vi "Populate Ring.vi"(5 "Sort Alphabetically instead of by Hierarchy?(T)":bool=TRUE, 7 "Close Reference?(T)":bool=TRUE, 8 "error in (no error)":errorcluster, 10 "Hierarchy Filter(empty=all)":string, 11 "Ring in":refnum<vi>) -> (0 "error out":errorcluster, 1 "Success?":bool, 3 "Classes found":string[](array[string]))   [LabVIEW 2020, in "ClassLoader.lvlib"]
doc: "Populate a ring control with a the hierarchy loaded using the given Hierarchy Filter."
uses:
  ClassLoader.lvlib
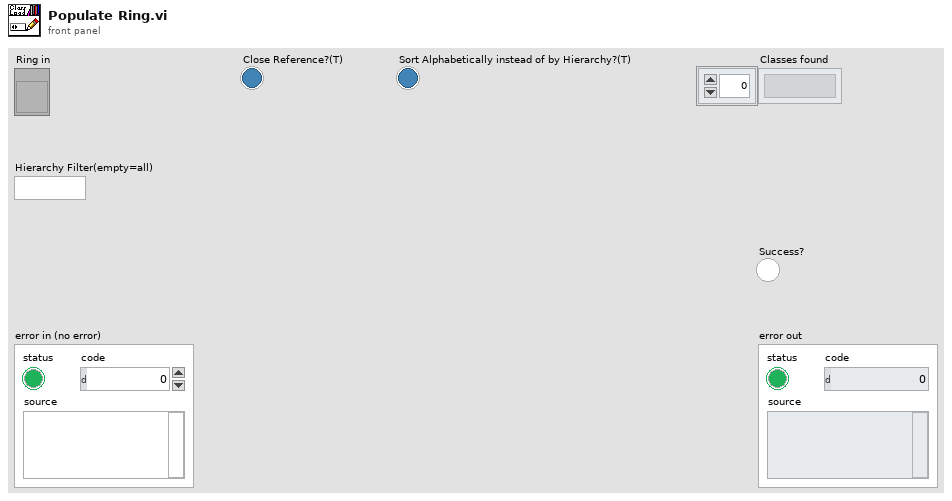
[diagram p1: front panel]
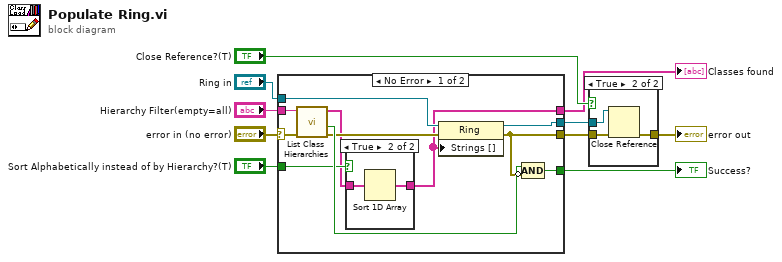
[diagram p0: block diagram]
diagram:
  n1 = case shown="No Error" "error in (no error)" {
    selector: "error in (no error)" -> [w18 w26]
    tunnel: [w21 _] -> w10
    tunnel: "Ring in" -> [w15 w25]
    tunnel: [w16 w25] -> w7
    tunnel: [w11 _] -> w6
    tunnel: "Hierarchy Filter(empty=all)" -> [w19 _]
    tunnel: [w13 w26] -> w3
    tunnel: "Sort Alphabetically instead of by Hierarchy?(T)" -> [w17 _]
    frame No Error {
      n2 = call "List Class Hierarchies.vi"("error in (no error)"=w18, "Hierarchy Filter(empty=all)"=w19) -> ("error out"=w14:errorcluster, "Success?"=w20:bool, "Classes found"=w12:string[])  [unwired: 6 in, 1 out]
      n3 = case shown="True" w17 {
        tunnel: [w22 w23] -> w11
        tunnel: w12 -> [w22 w24]
        frame False {
        }
        frame True {
          n4 = Sort 1D Array(array=w24) -> (sorted array=w23:string[])
        }
      }
      n5 = property class="Ring"(reference=w15, error in=w14, "Strings []"=w11) -> (reference out=w16:refnum<vi>, error out=w13:errorcluster)
      n6 = Compound Arithmetic op=AND(w20, invert w13) -> (w21:bool)
    }
    frame Error {
    }
  }
  "Success?" <- w10
  "Classes found" <- w6
  n7 = case shown="True" "Close Reference?(T)" {
    tunnel: w3 -> [w27 w30]
    tunnel: w7 -> [_ w29]
    tunnel: [w27 w28] -> w9
    frame False {
    }
    frame True {
      n8 = Close Reference(reference=w29, error in (no error)=w30) -> (error out=w28:errorcluster)
    }
  }
  "error out" <- w9
